vi "niScope Revision Query.vi"(0 "instrument handle":refnum<k15>, 11 "error in":errorcluster) -> (4 "instrument handle out":refnum<k15>, 6 "firmware revision":string, 10 "instrument driver revision":string, 15 "error out":errorcluster)   [LabVIEW 2013]
doc: "Returns the revision numbers of the instrument driver and instrument firmware."
uses:
  niScope_32.dll
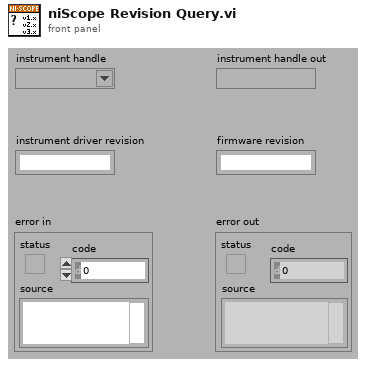
[diagram p1: front panel]
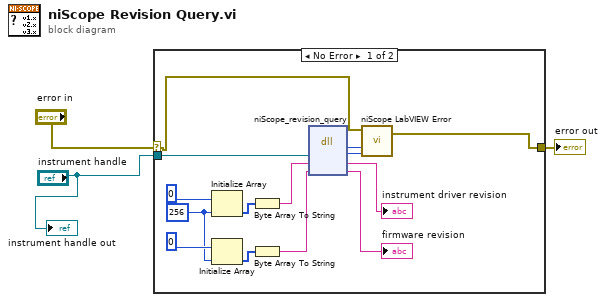
[diagram p0: block diagram]
diagram:
  n1 = case shown="No Error" "error in" {
    selector: "error in" -> [w4 w18]
    tunnel: [w5 w18] -> w3
    tunnel: "instrument handle" -> [w17 _]
    frame No Error {
      w8 = 256
      n2 = Initialize Array(u8 0, w8) -> (w15:u8[])
      n3 = Initialize Array(u8 0, w8) -> (w13:u8[])
      n4 = Byte Array To String(unsigned byte array=w15) -> (string=w12:string)
      n5 = Byte Array To String(unsigned byte array=w13) -> (string=w10:string)
      n6 = dll-call lib="niScope_*.*" fn="niScope_revision_query"("instrument handle"=w17, "instrumentDriverRevision"=w12, "firmwareRevision"=w10) -> ("status"=w6:i32, "instrument handle"=w7:u32, "instrumentDriverRevision"=→"instrument driver revision":string, "firmwareRevision"=→"firmware revision":string)  [unwired: 3 in, 2 out]
      n7 = call <instrlib>:"niScope LabVIEW Error.vi"("instrument handle"=w7, "niScope error code (0)"=w6, "error in (no error)"=w4) -> ("error out"=w5:errorcluster)  [unwired: 2 in]
    }
    frame Error {
    }
  }
  "error out" <- w3
  "instrument handle out" <- "instrument handle"
